vi "Initialize Instrument.vi"(8 "error in (no error)":errorcluster, 10 "Reset":bool, 11 "E3610x in":refnum<class "E3610x.lvclass">) -> (0 "error out":errorcluster, 3 "E3610x out":refnum<class "E3610x.lvclass">)   [LabVIEW 2020, in "E3610x.lvclass"]
uses:
  E3610x.lvclass
  C:/Sandbox/RF Bench/Source Code/WiSpry Test Framework/Instruments/Instrument.lvclass
  Instrument.lvclass/Instrument.ctl
  E3610x.lvclass/E3610x.ctl
  Power Supply.lvclass
  Instrument.lvclass
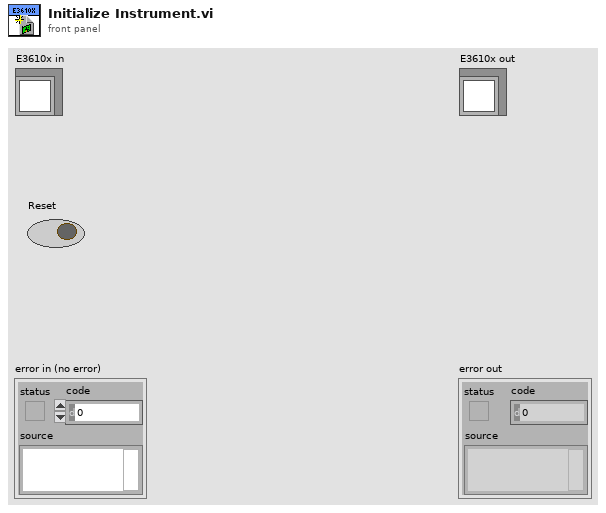
[diagram p1: front panel]
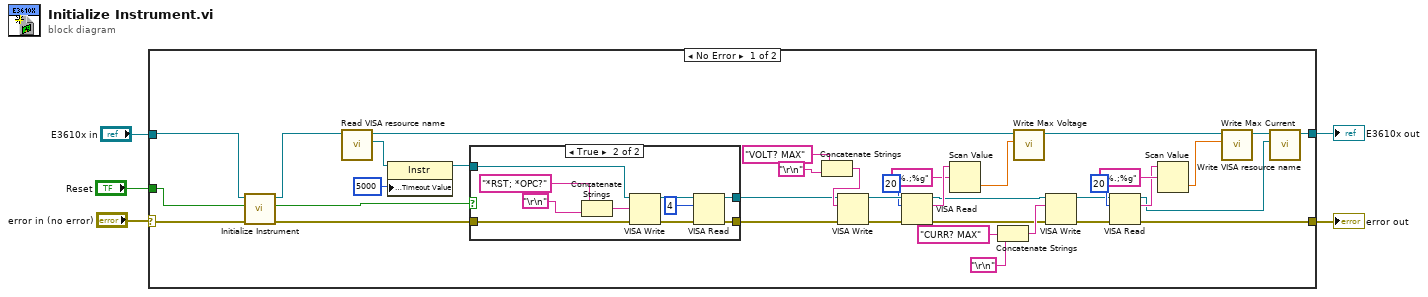
[diagram p0: block diagram]
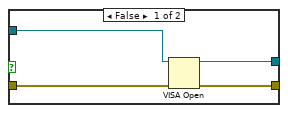
[diagram p2: hidden frame]
diagram:
  n1 = case shown="No Error" "error in (no error)" {
    selector: "error in (no error)" -> [w9 w56]
    tunnel: "E3610x in" -> [w7 w57]
    tunnel: "Reset" -> [w10 _]
    tunnel: [w14 w56] -> w2
    tunnel: [w41 w57] -> w1
    frame No Error {
      n2 = call-parent "Initialize Instrument.vi"("error in (no error)"=w9, "Reset"=w10, "Power Supply in"=w7) -> ("error out"=w8:errorcluster, "Power Supply out"=w6:refnum<class "E3610x.lvclass">)  [unwired: 7 in]
      n3 = call "Read VISA resource name.vi"("Instrument in"=w6) -> ("VISA resource name"=w12:refnum<visa-resource-name>, "Instrument out"=w30:refnum<class "E3610x.lvclass">)  [unwired: 9 in]
      n4 = property class="Instr"(reference=w12, "General Settings:Timeout Value"=u32 5000) -> (reference out=w11:refnum<visa-resource-name>)  [unwired: 1 in, 1 out]
      n5 = case shown="True" w10 {
        tunnel: w8 -> [w44 w55]
        tunnel: w11 -> [w45 w50]
        tunnel: [w42 w49] -> w37
        tunnel: [w43 w48] -> w36
        frame False {
          n6 = VISA Open(error in (no error)=w44, VISA resource name=w45) -> (VISA resource name=w42:refnum<visa-resource-name>, error out=w43:errorcluster)  [unwired: 3 in]
        }
        frame True {
          n7 = Concatenate Strings("*RST; *OPC?", "\r\n") -> (w47:string)
          n8 = VISA Write(VISA resource name=w50, write buffer=w47, error in (no error)=w55) -> (VISA resource name out=w52:refnum<visa-resource-name>, error out=w53:errorcluster)  [unwired: 1 out]
          n9 = VISA Read(VISA resource name=w52, byte count=u32 4, error in (no error)=w53) -> (VISA resource name out=w49:refnum<visa-resource-name>, error out=w48:errorcluster)  [unwired: 2 out]
        }
      }
      n10 = Concatenate Strings("VOLT? MAX", "\r\n") -> (w38:string)
      n11 = VISA Write(VISA resource name=w37, write buffer=w38, error in (no error)=w36) -> (VISA resource name out=w34:refnum<visa-resource-name>, error out=w35:errorcluster)  [unwired: 1 out]
      n12 = VISA Read(VISA resource name=w34, byte count=u32 20, error in (no error)=w35) -> (VISA resource name out=w17:refnum<visa-resource-name>, read buffer=w32:string, error out=w18:errorcluster)  [unwired: 1 out]
      n13 = Scan Value(string=w32, format string="%.;%g") -> (value=w29:dbl)  [unwired: 1 in, 1 out]
      n14 = Concatenate Strings("CURR? MAX", "\r\n") -> (w21:string)
      n15 = call "Write Max Voltage.vi"("Max Voltage"=w29, "E3610x in"=w30) -> ("E3610x out"=w28:refnum<class "E3610x.lvclass">)  [unwired: 9 in]
      n16 = VISA Write(VISA resource name=w17, write buffer=w21, error in (no error)=w18) -> (VISA resource name out=w23:refnum<visa-resource-name>, error out=w22:errorcluster)  [unwired: 1 out]
      n17 = VISA Read(VISA resource name=w23, byte count=u32 20, error in (no error)=w22) -> (VISA resource name out=w15:refnum<visa-resource-name>, read buffer=w25:string, error out=w14:errorcluster)  [unwired: 1 out]
      n18 = Scan Value(string=w25, format string="%.;%g") -> (value=w16:dbl)  [unwired: 1 in, 1 out]
      n19 = call "Write Max Current.vi"("Max Current"=w16, "E3610x in"=w28) -> ("E3610x out"=w27:refnum<class "E3610x.lvclass">)  [unwired: 9 in]
      n20 = call "Write VISA resource name.vi"("VISA resource name"=w15, "Instrument in"=w27) -> ("Instrument out"=w41:refnum<class "E3610x.lvclass">)  [unwired: 9 in]
    }
    frame Error {
    }
  }
  "error out" <- w2
  "E3610x out" <- w1
